vi "Identify.vi"(8 "error in (no error)":errorcluster, 11 "BML_LS Pattern Creator in":refnum<class "BML_LS Pattern Creator.lvclass">) -> (0 "error out":errorcluster, 2 "Plugin is Valid":bool, 3 "BML_LS Pattern Creator out":refnum<class "BML_LS Pattern Creator.lvclass">)   [LabVIEW 2018, in "BML_LS Pattern Creator.lvlib" / "BML_LS Pattern Creator.lvclass"]
uses:
  BML_LS Pattern Creator.lvclass
  C:/P4 Workspace/PC Client/Solutions/5g_eap/trunk/1.0/HiSi5GmmWave/Pattern_Gen_Tool/Interfaces/Protocol Interface.lvlibp/Interfaces/Protocol Interface/Protocol Interface.lvclass
  Interfaces/Protocol Interface.lvlibp/Ctls/Protocol Type.ctl
  Interfaces/Protocol Interface.lvlibp/Interfaces/Protocol Interface/Read Protocol Type.vi
  Interfaces/Protocol Interface.lvlibp
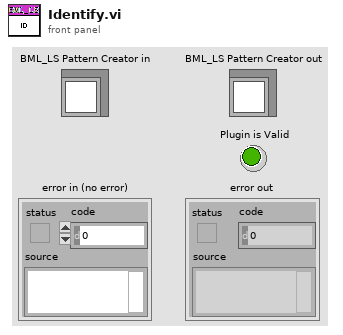
[diagram p1: front panel]
types:
  T1 = typedef "Protocol Interface.lvlibp/Protocol Type.ctl" = enum16{"BML_LS", "BML_HS", "SPI_3W", "SPI_4W"}
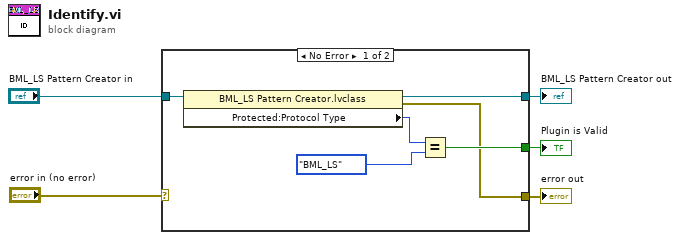
[diagram p0: block diagram]
diagram:
  n1 = case shown="No Error" "error in (no error)" {
    selector: "error in (no error)" -> [_ w12]
    tunnel: "BML_LS Pattern Creator in" -> [w11 w13]
    tunnel: [w8 _] -> w3
    tunnel: [w7 w13] -> w2
    tunnel: [w6 w12] -> w1
    frame No Error {
      n2 = property class="BML_LS Pattern Creator.lvclass"(reference=w11) -> (reference out=w7:refnum<class "BML_LS Pattern Creator.lvclass">, error out=w6:errorcluster, "Protected:Protocol Type"=w10:T1)  [unwired: 1 in]
      n3 = Equal?(x=w10, y=Protocol_Type."BML_LS") -> (x = y?=w8:bool)
    }
    frame Error {
    }
  }
  "error out" <- w1
  "BML_LS Pattern Creator out" <- w2
  "Plugin is Valid" <- w3
